vi "Stop Process.vi"(8 "error in (no error)":errorcluster, 11 "CoolApp in":refnum<class "CoolApp.lvclass">) -> (0 "error out":errorcluster, 3 "CoolApp out":refnum<class "CoolApp.lvclass">)   [LabVIEW 2020, in "LAF2024Q2.lvlib" / "CoolApp.lvclass"]
uses:
  CoolApp.lvclass
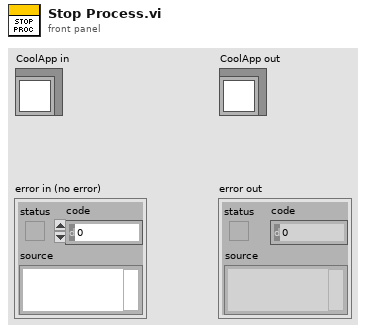
[diagram p1: front panel]
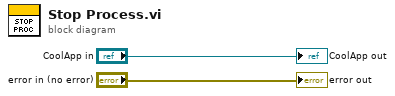
[diagram p0: block diagram]
diagram:
  "error out" <- "error in (no error)"
  "CoolApp out" <- "CoolApp in"
